vi "LimeSDR_FM_Tx_LabVIEW.vi"() -> ()   [LabVIEW 2018, in "LMS_LV_Drv.lvlib"]
uses:
  LMS_LV_Drv.lvlib
  <vilib>/addons/Modulation/Analog/support/mod_FM CE Modulation.vi
  <vilib>/addons/Modulation/niAMT.lvlib
  <vilib>/measure/NI_MABase.lvlib
panel:
  out "x*y":dbl=2525000.0
  in  "FM Deviation [Hz]":dbl=100000.0 format="%#.4p"
  in  "Message Frequency [Hz]":dbl=1000.0 format="%#_6p"
  in  "Signal type":T1(ring)
  out "unsigned 64bit integer":u64=2000000
  in  "Boolean":bool
  out "Numeric":i32=2022082730
  out "return":i32=2098176
  in  "Direction":u8(ring) items=["RX", "TX"]
  out "EXIT":bool=TRUE
  in  "stop":bool
  in  "FM  Frequency":dbl(slide)=100000000.0 min=85000000.0 max=108000000.0 step=50000.0 scale=85000000.0..108000000.0 scale format="%#_6p"
  in  "chan":u64
  out "LimeSDR_info":string="LimeSDR-USB, media=USB 3.0, module=FX3, serial=0009072C02891115, index=0"
  in  "Sample Rate":dbl=2000000.0 format="%#_6p"
  out "error out":errorcluster
  # "Two Tone Generation Demo"
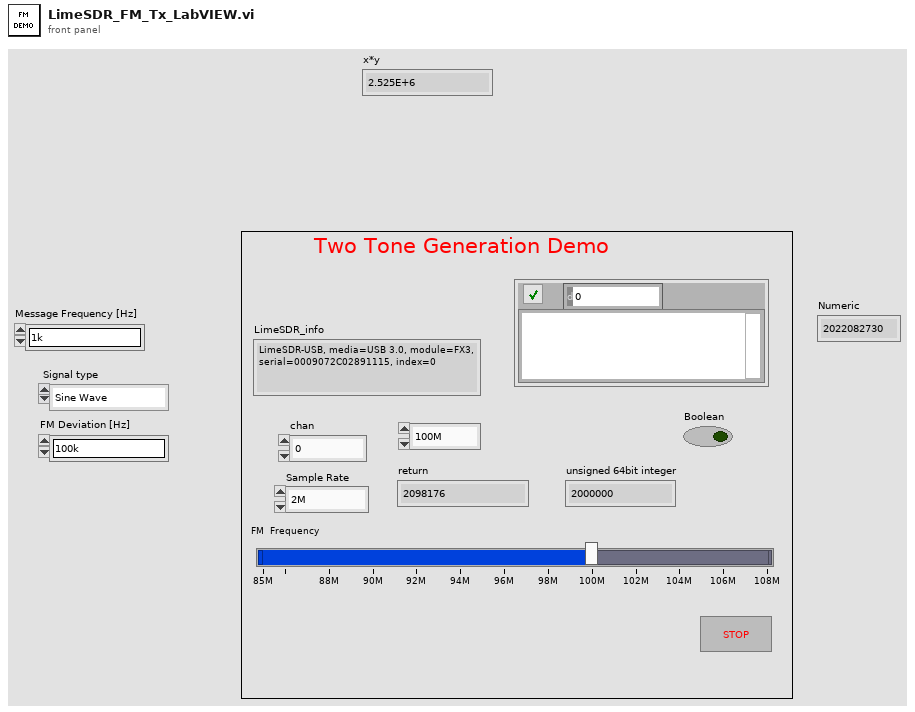
[diagram p1: front panel]
types:
  T1 = enum16{"Sine Wave", "Triangle Wave", "Square Wave", "Sawtooth Wave"}
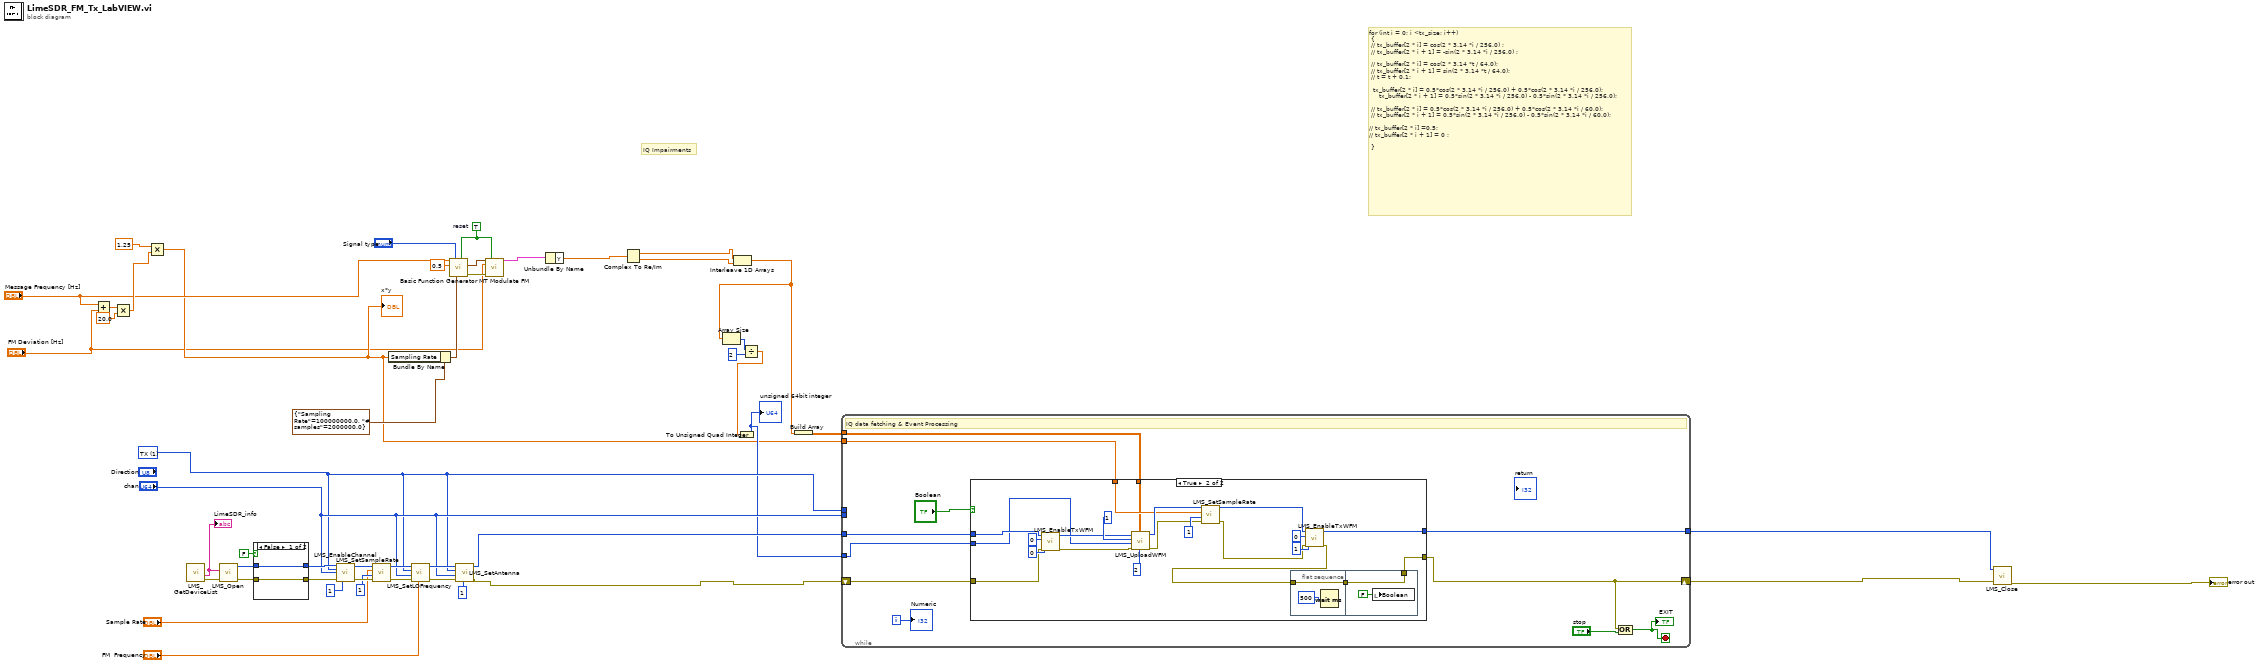
[diagram p0: block diagram]
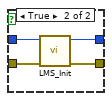
[diagram p2: hidden frame]
diagram:
  w14 = TRUE  # reset
  w32 = u8 1 items=["RX", "TX"] ("Direction")
  # "IQ Impairments"
  # "for (int i = 0; i <tx_size; i++)\n\t{\n\t//\ttx_buffer[2 * i] = cos(2 * 3.14 *i / 256.0) ;\n\t//\ttx_buffer[2 * i + 1] = -sin(2 * 3.14 *i / 256.0) ;\n\n\t//\ttx_buffer[2 * i] = cos(2 * 3.14 *t / 64.0);\n\t//\ttx_buffer[2 * i + 1] = sin(2 * 3.14 *t / 64.0);\n\t//\tt = t + 0.1;\n\n\t\ttx_buffer[2 * i] = 0.5*cos(2 * 3.14 *i / 256.0) + 0.5*cos(2 * 3.14 *i / 256.0);\n    \ttx_buffer[2 * i + 1] = 0.5*sin(2 * 3.14 *i / 256.0) - 0.5*sin(2 * 3.14 *i / 256.0);\n\n\t//\ttx_buffer[2 * i] = 0.5*cos(2 * 3.14 *i / 256.0) + 0.5*cos(2 * 3.14 *i / 60.0);\n\t//\ttx_buffer[2 * i + 1] = 0.5*sin(2 * 3.14 *i / 256.0) - 0.5*sin(2 * 3.14 *i / 60.0);\n\n//\ttx_buffer[2 * i] =0.5;\n//\ttx_buffer[2 * i + 1] = 0 ;\n\n\t}"
  n1 = Add(x="Message Frequency [Hz]", y="FM Deviation [Hz]") -> (x+y=w11:dbl)
  n2 = Multiply(x=w11, y=20.0) -> (x*y=w8:dbl)
  n3 = Multiply(x=1.25, y=w8) -> (x*y=w4:dbl)
  "x*y" <- w4
  n4 = call "LMS_GetDeviceList.vi"() -> ("error out"=w49:errorcluster, "lms_info_str_t"=w48:string)  [unwired: 9 in, 1 out]
  "LimeSDR_info" <- w48
  n5 = call "LMS_Open.vi"("error in (no error)"=w49, "lms_info_str_t"=w48) -> ("error out"=w47:errorcluster, "device"=w46:i64)  [unwired: 8 in]
  n6 = case shown="False" FALSE {
    tunnel: w47 -> [w50 w55]
    tunnel: w46 -> [w51 w54]
    tunnel: [w51 w53] -> w45
    tunnel: [w50 w52] -> w44
    frame False {
    }
    frame True {
      n7 = call "LMS_Init.vi"("error in (no error)"=w55, "device_In"=w54) -> ("error out"=w52:errorcluster, "device_Out"=w53:i64)  [unwired: 8 in]
    }
  }
  n8 = call "LMS_EnableChannel.vi"("device_In"=w45, "dir_tx"=w32, "chan"="chan", "error in (no error)"=w44, "enabled"=i8 1) -> ("device_Out"=w41:i64, "error out"=w42:errorcluster)  [unwired: 9 in]
  n9 = call "LMS_SetSampleRate.vi"("error in (no error)"=w42, "oversample"=u64 1, "rate"="Sample Rate", "device_In"=w41) -> ("error out"=w40:errorcluster, "device_Out"=w39:i64)  [unwired: 6 in]
  n10 = Bundle By Name(cluster=cluster{"Sampling Rate":dbl, "# samples":dbl} {"Sampling Rate"=100000000.0, "# samples"=2000000.0} ("sampling info"), "Sampling Rate"=w4) -> (w6:cluster{"Sampling Rate":dbl, "# samples":dbl})
  n11 = call "LMS_SetLOFrequency.vi"("frequency"="FM  Frequency", "error in (no error)"=w40, "chan"="chan", "dir_tx"=w32, "device_In"=w39) -> ("error out"=w37:errorcluster, "device_Out"=w36:i64)  [unwired: 5 in]
  n12 = call <vilib>:"Basic Function Generator.vi"("reset signal"=w14, "sampling info"=w6, "signal type"="Signal type", "amplitude"=0.5, "frequency"="Message Frequency [Hz]") -> ("error out"=w16:errorcluster, "signal out"=w15:waveform(dbl))  [unwired: 4 in, 1 out]
  n13 = call "LMS_SetAntenna.vi"("index"=u64 1, "error in (no error)"=w37, "chan"="chan", "dir_tx"=w32, "device_In"=w36) -> ("error out"=w29:errorcluster, "device_Out"=w27:i64)  [unwired: 5 in]
  n14 = call <vilib>:"MT Modulate FM.vi"("message signal"=w15, "reset? (F)"=w14, "FM deviation (Hz)"="FM Deviation [Hz]", "error in (no error)"=w16) -> ("FM modulated waveform"=w12:cluster{"t0":dbl, "dt":dbl, "Y":cdb[]})  [unwired: 10 in, 1 out]
  n15 = Unbundle By Name(w12) -> ("Y"=w22:cdb[])
  n16 = Complex To Re/Im(x + iy=w22) -> (x=w24:dbl[], y=w23:dbl[])
  n17 = Interleave 1D Arrays(w24, w23) -> (w21:dbl[])
  n18 = Array Size(array=w21) -> (size(s)=w20:i32)
  n19 = Divide(x=w20, y=2) -> (x/y=w18:dbl)
  n20 = To Unsigned Quad Integer(1:w18) -> (0:w17:u64)
  "unsigned 64bit integer" <- w17
  n21 = Build Array(w21) -> (w25:dbl[][])
  n22 = while {
    shift-right: [w62] -> w28
    shift-left: w29 -> [w63]
    tunnel: w32 -> [_]
    tunnel: "chan" -> [_]
    tunnel: w17 -> [w58]
    tunnel: w27 -> [w61]
    tunnel: [w60] -> w26
    tunnel: w25 -> [w59]
    tunnel: w4 -> [w56]
    i -> [w64]
    stop <- w66 stop-if-true
    # "IQ data fetching & Event Processing"
    n23 = case shown="True" "Boolean" {
      tunnel: w63 -> [w67 w80]
      tunnel: [w67 w85] -> w62
      tunnel: w61 -> [w68 w77]
      tunnel: [w68 w90] -> w60
      tunnel: w59 -> [_ w69]
      tunnel: w58 -> [_ w76]
      tunnel: w56 -> [_ w70]
      frame False {
      }
      frame True {
        n24 = call "LMS_EnableTxWFM.vi"("error in (no error)"=w80, "active"=i8 0, "chan"=u64 0, "device_In"=w77) -> ("error out"=w79:errorcluster, "device_Out"=w78:i64)  [unwired: 6 in]
        n25 = call "LMS_UploadWFM.vi"("format"=2, "samples"=w69, "error in (no error)"=w79, "sample_count"=w76, "ChannelCount"=u8 1, "Dev"=w78) -> ("error out"=w72:errorcluster, "Dev_out"=w74:i64)  [unwired: 4 in]
        n26 = call "LMS_SetSampleRate.vi"("error in (no error)"=w72, "oversample"=u64 1, "rate"=w70, "device_In"=w74) -> ("error out"=w71:errorcluster, "device_Out"=w73:i64)  [unwired: 6 in]
        n27 = flat-sequence {
          tunnel: [w91] -> w84
          tunnel: w83 -> [w91]
          tunnel: [w93] -> w85
          tunnel: w84 -> [w93]
          frame #0 {
            n28 = Wait (ms)(milliseconds to wait=u32 500) -> ()  [unwired: 1 out]
          }
          frame #1 {
            n29 = local write "Boolean"(FALSE ("Boolean")) -> ()
          }
        }
        n30 = call "LMS_EnableTxWFM.vi"("error in (no error)"=w71, "active"=i8 1, "chan"=u64 0, "device_In"=w73) -> ("error out"=w83:errorcluster, "device_Out"=w90:i64)  [unwired: 6 in]
      }
    }
    n31 = Compound Arithmetic op=OR(w62, "stop") -> (w66:bool)
    "EXIT" <- w66
    "Numeric" <- w64
  }
  n32 = call "LMS_Close.vi"("error in (no error)"=w28, "device_In"=w26) -> ("error out"=→"error out":errorcluster)  [unwired: 9 in]
